vi "Initialize Event Registrations.vi"(8 "error in (no error)":errorcluster, 11 "Events-References":T1) -> (0 "error out":errorcluster, 3 "Event-Registrations":T2)   [LabVIEW 2018, in "Actor.lvclass"]
uses:
  Actor.lvclass
  Event-Registrations.ctl
  Stop.ctl
  Event-References.ctl
  Actor Class Launched.ctl
  Example-Request.ctl
  Example-Reply.ctl
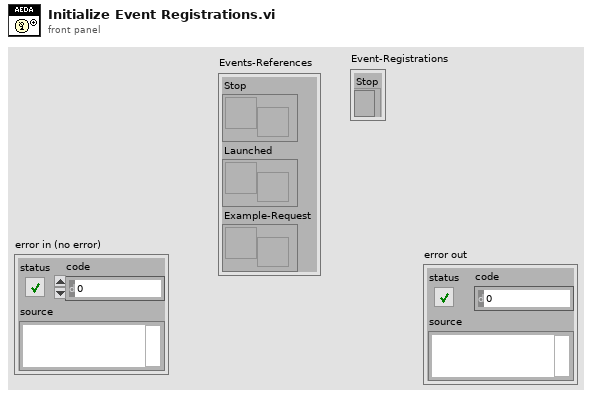
[diagram p1: front panel]
types:
  T1 = typedef "Actor.lvclass/Event-References.ctl" = cluster{"Stop":refnum<user-event>, "Launched":refnum<user-event>, "Example-Request":refnum<user-event>}
  T2 = typedef "Actor.lvclass/Event-Registrations.ctl" = cluster{"Stop":refnum<event-registration>}
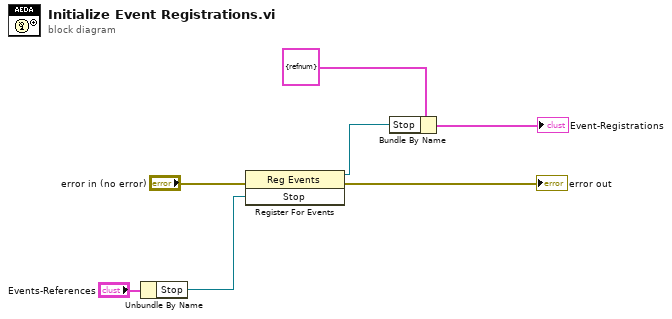
[diagram p0: block diagram]
diagram:
  n1 = Unbundle By Name("Events-References") -> ("Stop"=w4:refnum<user-event>)
  n2 = register-events(error in="error in (no error)", w4) -> (reference out=w3:refnum<event-registration>, error out=→"error out":errorcluster)  [unwired: 1 in]
  n3 = Bundle By Name(cluster=T2 {"Stop"=refnum} ("Actor-Event-Registrations"), "Stop"=w3) -> (→"Event-Registrations":T2)
